vi "SetProcessVersion.vi"(8 "error in":errorcluster, 10 "ProcessVersion":string, 11 "OperationCycle in":refnum<class "OperationCycle.lvclass">) -> (0 "error out":errorcluster, 3 "OperationCycle out":refnum<class "OperationCycle.lvclass">)   [LabVIEW 2021, in "ProligentXMLGenerator.lvlib" / "OperationCycle.lvclass"]
doc: "Defines the process version of the process in which this operation run is defined. This field is optional to support non-versionable processes. The version string must be string-comparable to support ordering by version.\n\nThis attribute cannot be updated."
uses:
  OperationCycle.lvclass
  OperationCycle.lvclass/OperationCycle.ctl
  Base/Attribute/Attribute.lvclass
  Base/NonEmptyString_64/NonEmptyString_64.lvclass
  C:/Projects/proligent-xml-generator-labview/src/ProligentXMLGenerator/Base/NonEmptyString/NonEmptyString.lvclass
  C:/Projects/proligent-xml-generator-labview/src/ProligentXMLGenerator/Base/String/String.lvclass
  C:/Projects/proligent-xml-generator-labview/src/ProligentXMLGenerator/Base/Attribute/Attribute.lvclass
  C:/Projects/proligent-xml-generator-labview/src/ProligentXMLGenerator/Base/NonEmptyString_64/NonEmptyString_64.lvclass
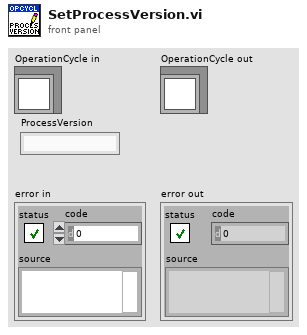
[diagram p1: front panel]
types:
  T1 = typedef "ProligentXMLGenerator.lvlib/OperationCycle.lvclass/Data.ctl" = cluster{"Name":string, "CustomData":refnum<class "CustomData.lvclass">, "ProcessFullName":refnum<class "ProcessFullName.lvclass">, "ProcessVersion":refnum<class "NonEmptyString_64.lvclass">, "OperationCycleId":refnum<class "Guid.lvclass">, "OperationName":refnum<class "NonEmptyString_65.lvclass">, "Location":refnum<class "FullName.lvclass">, "User":refnum<class "NonEmptyString_255.lvclass">, "OperationCycleStatus":refnum<class "ExecutionStatus.lvclass">, "OperationCycleStartTime":refnum<class "DateTime.lvclass">, "OperationCycleEndTime":refnum<class "DateTime.lvclass">, "TimeZoneInfoId":string}
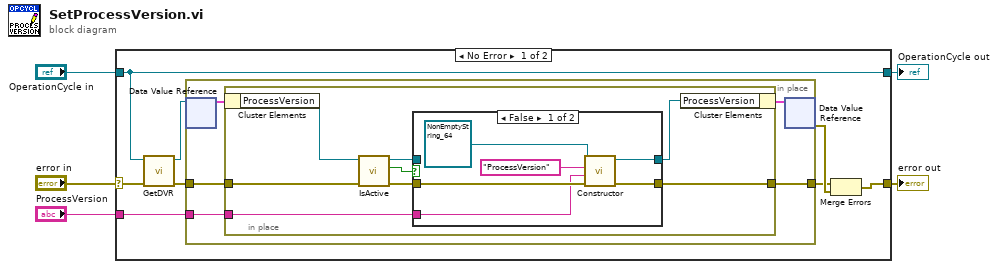
[diagram p0: block diagram]
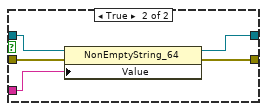
[diagram p2: hidden frame]
diagram:
  n1 = case shown="No Error" "error in" {
    selector: "error in" -> [w11 w38]
    tunnel: "OperationCycle in" -> [w6 w39]
    tunnel: [w8 w38] -> w3
    tunnel: "ProcessVersion" -> [w7 _]
    tunnel: [w6 w39] -> w1
    frame No Error {
      n2 = call "GetDVR.vi"("error in"=w11, "OperationCycle in"=w6) -> ("error out"=w10:errorcluster, "DVRReference"=w12:refnum<data-value>)  [unwired: 8 in]
      n3 = in-place "In Place Element Structure" {
        in-place-border: w10 -> [w18]
        in-place-border: [w17] -> w9
        in-place-border: w7 -> [w16]
        n4 = in-place-dvr #1(w12) -> (w15:T1)  [unwired: 1 out]
        n5 = in-place "In Place Element Structure" {
          in-place-border: w18 -> [w22]
          in-place-border: [w26] -> w17
          in-place-border: w16 -> [w25]
          n6 = in-place-cluster #2(w15) -> ("ProcessVersion"=w21:refnum<class "NonEmptyString_64.lvclass">)
          n7 = call "IsActive.vi"("error in"=w22, "Attribute in"=w21) -> ("error out"=w23:errorcluster, "IsActive"=w19:bool, "Attribute in"=w20:refnum<class "NonEmptyString_64.lvclass">)  [unwired: 7 in]
          n8 = case shown="False" w19 {
            tunnel: w23 -> [w29 w37]
            tunnel: [w32 w36] -> w26
            tunnel: w25 -> [w28 w35]
            tunnel: [w31 w34] -> w24
            tunnel: w20 -> [_ w33]
            frame False {
              n9 = call-dynamic "Constructor.vi"("error in"=w29, "Value"=w28, "Name"="ProcessVersion", "String in"=refnum<class "NonEmptyString_64.lvclass"> refnum ("ProcessVersion")) -> ("error out"=w32:errorcluster, "String out"=w31:refnum<class "NonEmptyString_64.lvclass">)  [unwired: 6 in]
            }
            frame True {
              n10 = property on="Property Node" class="NonEmptyString_64"(reference=w33, error in=w37, "Value"=w35) -> (reference out=w34:refnum<class "NonEmptyString_64.lvclass">, error out=w36:errorcluster)
            }
          }
          n11 = in-place-cluster #2("ProcessVersion"=w24) -> (w14:T1)
        }
        n12 = in-place-dvr #1(w14) -> (w13:errorcluster)  [unwired: 1 out]
      }
      n13 = Merge Errors(w9, w13) -> (w8:errorcluster)
    }
    frame Error {
    }
  }
  "error out" <- w3
  "OperationCycle out" <- w1
